vi "Update Template Files.vi"(8 "error in (no error)":errorcluster, 11 "Server Library (Library Item) in":refnum<vi>) -> (0 "error out":errorcluster, 3 "Server Library (Library Item) out":refnum<vi>)   [LabVIEW 2019, in "gRPC Scripting Tools.lvlib"]
uses:
  gRPC Scripting Tools.lvlib
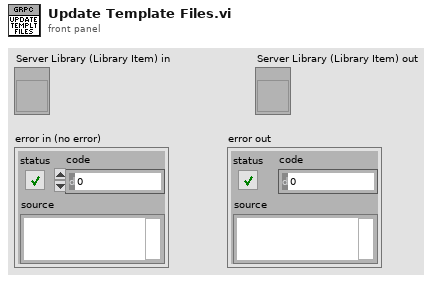
[diagram p1: front panel]
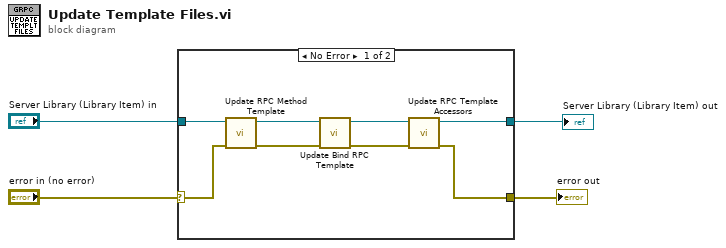
[diagram p0: block diagram]
diagram:
  n1 = case shown="No Error" "error in (no error)" {
    selector: "error in (no error)" -> [w11 w14]
    tunnel: "Server Library (Library Item) in" -> [w12 w13]
    tunnel: [w6 w14] -> w2
    tunnel: [w5 w13] -> w1
    frame No Error {
      n2 = call "Update RPC Method Template.vi"("error in (no error)"=w11, "Server Library (Library Item) in"=w12) -> ("error out"=w10:errorcluster, "Server Library (Library Item) out"=w9:refnum<vi>)  [unwired: 8 in]
      n3 = call "Update Bind RPC Template.vi"("error in (no error)"=w10, "Server Library (Library Item) in"=w9) -> ("error out"=w8:errorcluster, "Server Library (Library Item) out"=w7:refnum<vi>)  [unwired: 8 in]
      n4 = call "Update RPC Template Accessors.vi"("error in (no error)"=w8, "Server Library (Library Item) in"=w7) -> ("error out"=w6:errorcluster, "Server Library (Library Item) out"=w5:refnum<vi>)  [unwired: 8 in]
    }
    frame Error {
    }
  }
  "Server Library (Library Item) out" <- w1
  "error out" <- w2
